vi "GetCurrentState.vi"(9 "error in (no error)":errorcluster, 11 "States":cluster{"Current State":T1, "Next States":T2}) -> (1 "error out":errorcluster, 3 "Current State":string)   [LabVIEW 2020, in "StateMachine.lvlib"]
uses:
  StateMachine.lvlib
  TDefs/State.ctl
  TDefs/States.ctl
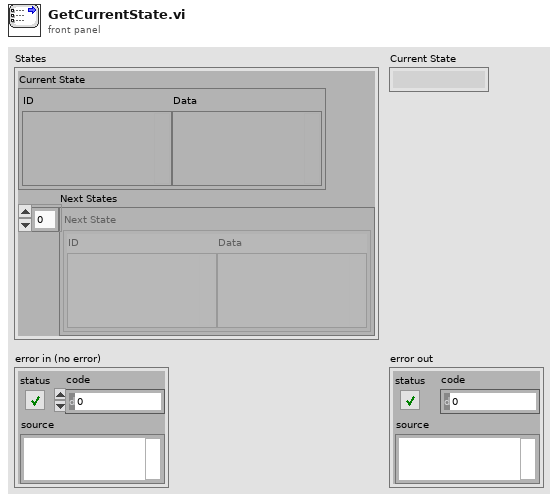
[diagram p1: front panel]
types:
  T1 = typedef "StateMachine.lvlib/State.ctl" = cluster{"ID":variant, "Data":variant}
  T2 = typedef "StateMachine.lvlib/States.ctl" = T1[]
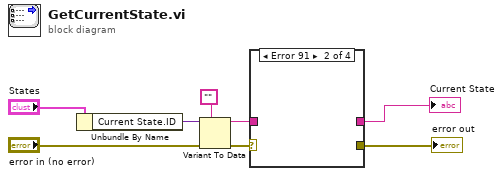
[diagram p0: block diagram]
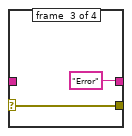
[diagram p3: hidden frame]
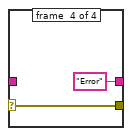
[diagram p4: hidden frame]
diagram:
  n1 = Unbundle By Name("States") -> ("Current State.ID"=w8:variant)
  n2 = Variant To Data(error in="error in (no error)", type="", Variant=w8) -> (data=w4:string, error out=w3:errorcluster)
  n3 = case shown="Error 91" w3 {
    selector: w3 -> [w9 _ w12 w14]
    tunnel: w4 -> [w10 _ _ _]
    tunnel: [w10 _ "Error" "Error"] -> w5
    tunnel: [w9 _ w12 w14] -> w6
    frame #0 {
    }
    frame #1 {
    }
    frame #2 {
    }
    frame #3 {
    }
  }
  "error out" <- w6
  "Current State" <- w5
